vi "Create Class Overview.vi"(8 "error in":errorcluster, 10 "Classes":refnum<class "Class.lvclass">[](array[class]), 11 "Uml":string) -> (0 "error out":errorcluster, 3 "Classes Overview out":refnum<class "Classes Overview.lvclass">)   [LabVIEW 2021, in "TAF Proj Document Type.lvlib" / "Classes Overview.lvclass"]
uses:
  <vilib>/Wovalab/AntiDoc/Document Type/Add-ons/LabVIEW TAF Project/Classes Overview/Classes Overview.lvclass
  C:/Program Files (x86)/National Instruments/LabVIEW 2021/vi.lib/Wovalab/AntiDoc/Bloc/Bloc.lvclass
  <vilib>/Wovalab/AntiDoc/Document Type/Add-ons/LabVIEW TAF Project/Class/Class.lvclass
  <vilib>/Wovalab/AntiDoc/Bloc/Bloc.lvclass/Bloc.ctl
  <vilib>/Wovalab/AntiDoc/Document Type/Add-ons/LabVIEW TAF Project/Classes Overview/Classes Overview.lvclass/Classes Overview.ctl
  <vilib>/Wovalab/AntiDoc/Bloc/Write Name.vi
  <vilib>/Wovalab/AntiDoc/Document Type/Add-ons/LabVIEW TAF Project/Classes Overview/Write Uml.vi
  <vilib>/Wovalab/AntiDoc/Document Type/Add-ons/LabVIEW TAF Project/Classes Overview/Write Classes.vi
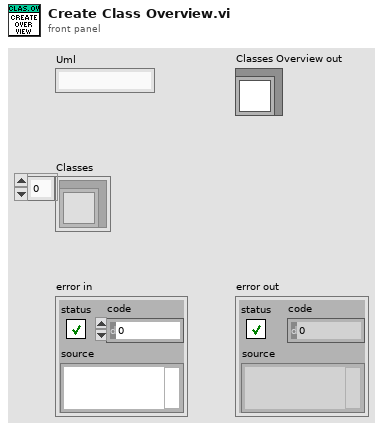
[diagram p1: front panel]
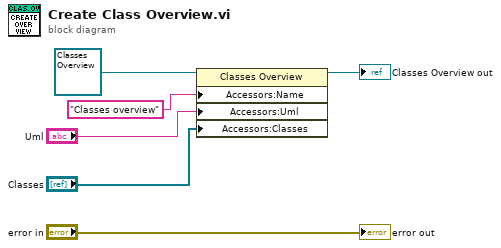
[diagram p0: block diagram]
diagram:
  n1 = property class="Classes Overview"(reference=refnum<class "Classes Overview.lvclass"> refnum ("Classes Overview in"), "Accessors:Name"="Classes overview" ("Title"), "Accessors:Uml"="Uml", "Accessors:Classes"="Classes") -> (reference out=→"Classes Overview out":refnum<class "Classes Overview.lvclass">)  [unwired: 1 in, 1 out]
  "error out" <- "error in"
